vi "Com_Matrix220_Release.vi"(8 "error in":errorcluster, 11 "Buffer Data":T1) -> (0 "error out":errorcluster)   [LabVIEW 2016]
uses:
  Data Def/Com_Matrix220_Buffer Data.ctl
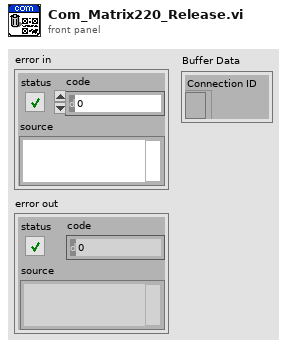
[diagram p1: front panel]
types:
  T1 = typedef "Com_Matrix220_Buffer Data.ctl" = cluster{"Connection ID":refnum<k5>}
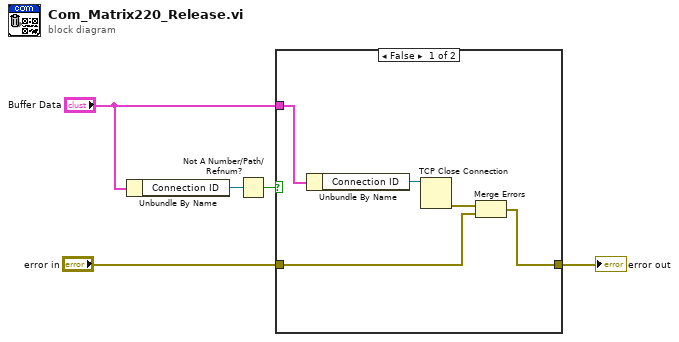
[diagram p0: block diagram]
diagram:
  n1 = Unbundle By Name("Buffer Data") -> ("Connection ID"=w5:refnum<k5>)
  n2 = Not A Number/Path/Refnum?(number/path/refnum=w5) -> (NaN/Path/Refnum?=w4:bool)
  n3 = case shown="False" w4 {
    tunnel: "Buffer Data" -> [w10 _]
    tunnel: "error in" -> [w7 w11]
    tunnel: [w6 w11] -> w1
    frame False {
      n4 = Unbundle By Name(w10) -> ("Connection ID"=w9:refnum<k5>)
      n5 = TCP Close Connection(connection ID=w9) -> (error out=w8:errorcluster)  [unwired: 2 in, 1 out]
      n6 = Merge Errors(w8, w7) -> (w6:errorcluster)
    }
    frame True {
    }
  }
  "error out" <- w1
